vi "Change AO Chan Gain on Fly (24bit).vi"(8 "error in (no error)":errorcluster, 9 "Gain Setting":u16(ring) items=["0 dB Gain"=0, "20 dB Gain"=2, "40 dB Gain"=4], 10 "channel":string="AO01") -> (0 "error out":errorcluster)   [LabVIEW 2015]
uses:
  PXI Globals.vi
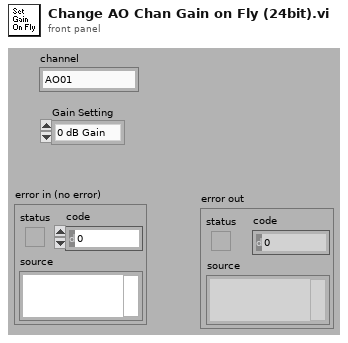
[diagram p1: front panel]
types:
  T1 = typedef "Task Struct.ctl" = cluster{"Task name":string, "Task":refnum<k21>, "Dual-channel task?":bool, "Regenerate?":bool, "Clear?":bool}
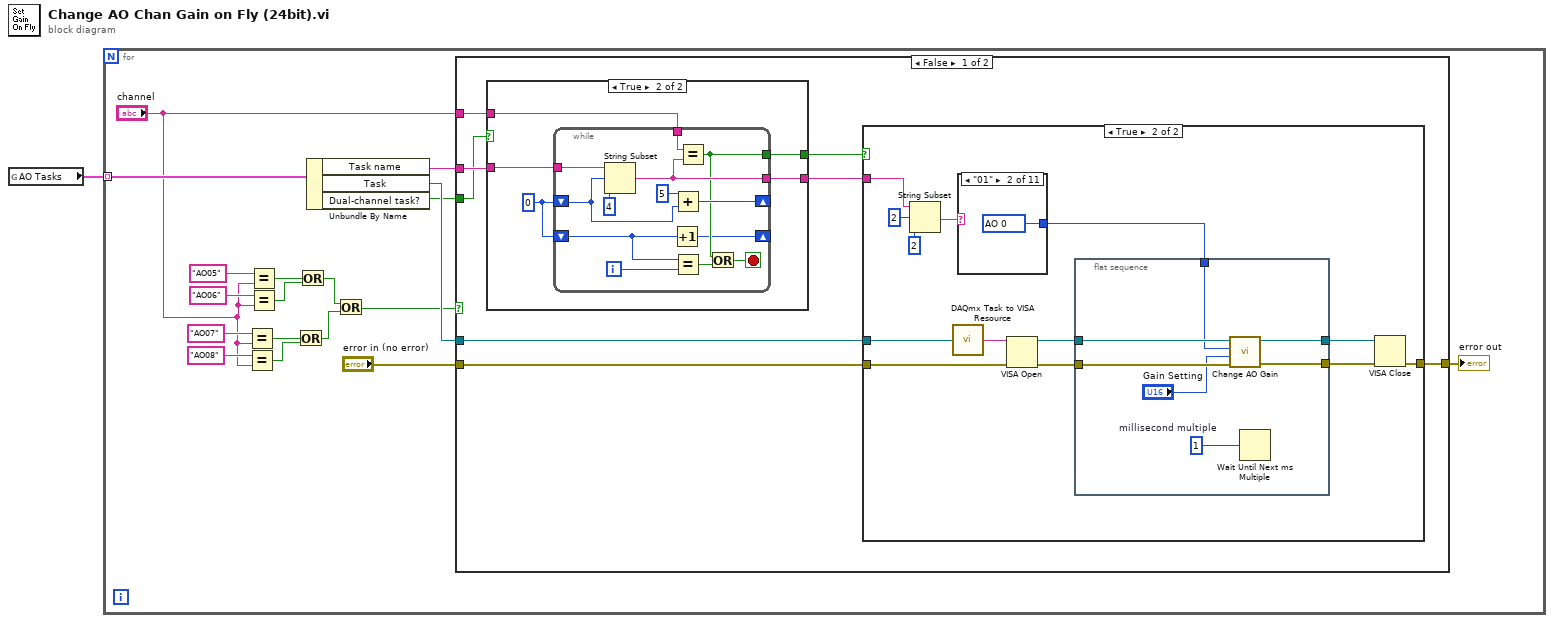
[diagram p0: block diagram]
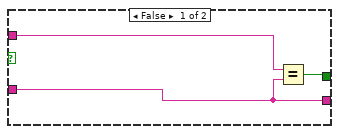
[diagram p2: hidden frame]
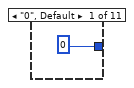
[diagram p4: hidden frame]
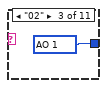
[diagram p5: hidden frame]
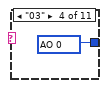
[diagram p6: hidden frame]
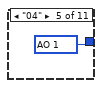
[diagram p7: hidden frame]
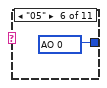
[diagram p8: hidden frame]
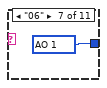
[diagram p9: hidden frame]
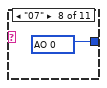
[diagram p10: hidden frame]
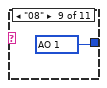
[diagram p11: hidden frame]
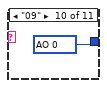
[diagram p12: hidden frame]
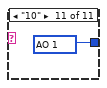
[diagram p13: hidden frame]
diagram:
  n1 = global read "PXI Globals.vi" "AO Tasks"() -> (w1:T1[])
  n2 = for {
    tunnel: w1 -> [w19] mode=indexing
    n3 = Equal?(x="AO07" ("Local Terminal Name"), y="channel") -> (x = y?=w8:bool)
    n4 = Equal?(x="AO08" ("Local Terminal Name"), y="channel") -> (x = y?=w9:bool)
    n5 = Equal?(x="AO05" ("Local Terminal Name"), y="channel") -> (x = y?=w12:bool)
    n6 = Equal?(x="AO06" ("Local Terminal Name"), y="channel") -> (x = y?=w13:bool)
    n7 = Or(x=w8, y=w9) -> (x .or. y?=w5:bool)
    n8 = Or(x=w12, y=w13) -> (x .or. y?=w4:bool)
    n9 = Unbundle By Name(w19) -> ("Task name"=w15:string, "Task"=w16:refnum<k21>, "Dual-channel task?"=w14:bool)
    n10 = Or(x=w4, y=w5) -> (x .or. y?=w3:bool)
    n11 = case shown="False" w3 {
      tunnel: [w27 w81] -> w18
      tunnel: "error in (no error)" -> [w26 w81]
      tunnel: w16 -> [w25 _]
      tunnel: w15 -> [w24 _]
      tunnel: w14 -> [w23 _]
      tunnel: "channel" -> [w20 _]
      frame False {
        n12 = case shown="True" w23 {
          tunnel: w24 -> [w28 w35]
          tunnel: [w28 w34] -> w22
          tunnel: [w30 w33] -> w21
          tunnel: w20 -> [w29 w32]
          frame False {
            n13 = Equal?(x=w29, y=w28) -> (x = y?=w30:bool)
          }
          frame True {
            w31 = 0
            n14 = while {
              tunnel: w35 -> [w48]
              tunnel: [w43] -> w34
              shift-right: [w46] -> _
              shift-left: w31 -> [w44]
              tunnel: [w40] -> w33
              tunnel: w32 -> [w42]
              shift-right: [w39] -> _
              shift-left: w31 -> [w37]
              i -> [w36]
              stop <- w41 stop-if-true
              n15 = String Subset(string=w48, offset (0)=w44, length (rest)=4 ("length (rest)")) -> (substring=w43:string)
              n16 = Increment(x=w37) -> (x+1=w39:i32)
              n17 = Add(x=5, y=w44) -> (x+y=w46:i32)
              n18 = Equal?(x=w37, y=w36) -> (x = y?=w38:bool)
              n19 = Equal?(x=w42, y=w43) -> (x = y?=w40:bool)
              n20 = Or(x=w40, y=w38) -> (x .or. y?=w41:bool)
            }
          }
        }
        n21 = case shown="True" w21 {
          tunnel: w25 -> [_ w56]
          tunnel: [w49 w55] -> w27
          tunnel: w26 -> [w49 w54]
          tunnel: w22 -> [_ w50]
          frame False {
          }
          frame True {
            n22 = String Subset(string=w50, offset (0)=2, length (rest)=2 ("length (rest)")) -> (substring=w51:string)
            n23 = call "DAQmx Task to VISA Resource.vi"("task out"=w56) -> ("VISAName"=w62:string)
            n24 = case shown="\"01\"" w51 {
              tunnel: [0 w71 w72 w73 w74 w75 w76 w77 w78 w79 w80] -> w57
              frame "0", Default {
              }
              frame "01" {
                w71 = u16 1536 items=["AO 0"=1536, "AO 1"=1540] ("AO Channel")
              }
              frame "02" {
                w72 = u16 1540 items=["AO 0"=1536, "AO 1"=1540] ("AO Channel")
              }
              frame "03" {
                w73 = u16 1536 items=["AO 0"=1536, "AO 1"=1540] ("AO Channel")
              }
              frame "04" {
                w74 = u16 1540 items=["AO 0"=1536, "AO 1"=1540] ("AO Channel")
              }
              frame "05" {
                w75 = u16 1536 items=["AO 0"=1536, "AO 1"=1540] ("AO Channel")
              }
              frame "06" {
                w76 = u16 1540 items=["AO 0"=1536, "AO 1"=1540] ("AO Channel")
              }
              frame "07" {
                w77 = u16 1536 items=["AO 0"=1536, "AO 1"=1540] ("AO Channel")
              }
              frame "08" {
                w78 = u16 1540 items=["AO 0"=1536, "AO 1"=1540] ("AO Channel")
              }
              frame "09" {
                w79 = u16 1536 items=["AO 0"=1536, "AO 1"=1540] ("AO Channel")
              }
              frame "10" {
                w80 = u16 1540 items=["AO 0"=1536, "AO 1"=1540] ("AO Channel")
              }
            }
            n25 = VISA Open(error in (no error)=w54, VISA resource name=w62) -> (VISA resource name=w58:refnum<visa-resource-name>, error out=w59:errorcluster)  [unwired: 3 in]
            n26 = flat-sequence {
              tunnel: w58 -> [w69]
              tunnel: w59 -> [w68]
              tunnel: [w67] -> w60
              tunnel: [w66] -> w61
              tunnel: w57 -> [w63]
              frame #0 {
                w64 = u32 1  # millisecond multiple
                n27 = call "Change AO Gain.vi"("error in"=w68, "Gain Setting"="Gain Setting", "AO Channel"=w63, "VISA resource name 2"=w69) -> ("error out"=w66:errorcluster, "VISA resource name"=w67:refnum<visa-resource-name>)  [unwired: 4 in]
                n28 = Wait Until Next ms Multiple(millisecond multiple=w64) -> ()  [unwired: 1 out]
              }
            }
            n29 = VISA Close(VISA resource name=w60, error in (no error)=w61) -> (error out=w55:errorcluster)
          }
        }
      }
      frame True {
      }
    }
    "error out" <- w18
  }
